vi "translate.vi"(8 "error in (no error)":errorcluster, 11 "ImagingModeDL090130Frame in":refnum<class "ImagingModeDL090130Frame.lvclass">=refnum) -> (0 "error out":errorcluster, 3 "ImagingModeDL090130Frame out":refnum<class "ImagingModeDL090130Frame.lvclass">)   [LabVIEW 2010, in "ImagingModeDL090130Frame.lvclass"]
uses:
  ImagingModeDL090130Frame.lvclass
  ScanHead/GenericScanHead/GenericScanHead/GenericScanHead.lvclass
  common/classes/GenericComponent/GenericComponent/GenericComponent.lvclass
  Adapter/GenericAdapter/GenericAdapter/GenericAdapter.lvclass
  ImagingModeDL090130Frame.lvclass/ImagingModeDL090130Frame.ctl
  common/classes/ErrorController/ErrorController/class_data.vi
  common/classes/ErrorController/ErrorController/ErrorController.lvclass
  Stage/GenericStage/GenericStage/GenericStage.lvclass
  Stage/GenericStage/GenericStage/translation_mode_enum.ctl
  GenericImagingMode/GenericImagingMode/GenericImagingMode.lvclass
  common/classes/SpaceVector/SpaceVector/SpaceVector.lvclass
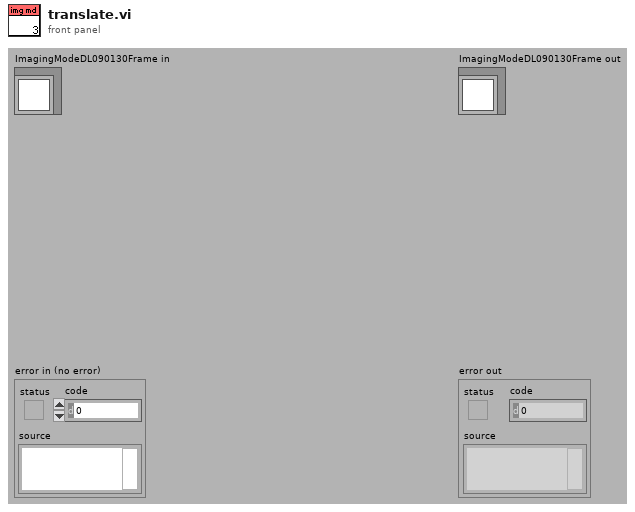
[diagram p1: front panel]
types:
  T1 = typedef "GenericStage.lvclass/translation_mode_enum.ctl" = enum16{"DON'T MOVE", "relative", "absolute"}
  T2 = typedef "ImagingModeDL090130Frame.lvclass/translation_mode_enum.ctl" = enum16{"scanHead", "stage"}
  T3 = typedef "GenericToplevelComponent.lvclass/common_trigger_enum.ctl" = enum16{"NULL", "initialise", "terminate", "fetch command", "fetch data", "attach observer", "register as observer", "detach observer", "acknowledge", "start", "stop", "sweep started", "sweep finished", "experiment started", "experiment stopped"}
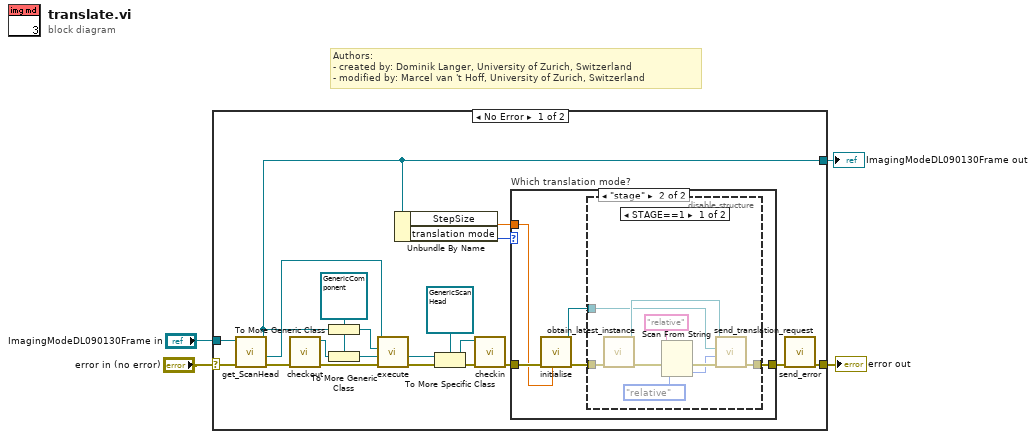
[diagram p0: block diagram]
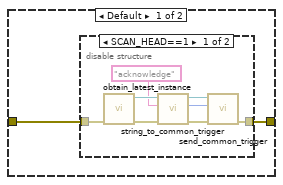
[diagram p2: hidden frame]
diagram:
  # "Authors: \n- created by: Dominik Langer, University of Zurich, Switzerland\n- modified by: Marcel van 't Hoff, University of Zurich, Switzerland"
  n1 = case shown="No Error" "error in (no error)" {
    selector: "error in (no error)" -> [w9 w52]
    tunnel: [w22 w52] -> w3
    tunnel: [w5 w51] -> w1
    tunnel: "ImagingModeDL090130Frame in" -> [w7 w51]
    frame No Error {
      w10 = refnum<class "GenericComponent.lvclass"> refnum ("GenericComponent.lvclass")
      n2 = call-dynamic "get_ScanHead.vi"("error in (no error)"=w9, "ScanModeDL090923Scaffold in"=w7) -> ("error out"=w8:errorcluster, "ScanHead adapter"=w6:refnum<class "GenericAdapter.lvclass">, "ScanModeDL090923Scaffold out"=w5:refnum<class "ImagingModeDL090130Frame.lvclass">)  [unwired: 4 in, 3 out]
      n3 = call "checkout.vi"("error in (no error)"=w8) -> ("error out"=w20:errorcluster, "GenericScanHead out"=w19:refnum<class "GenericScanHead.lvclass">)  [unwired: 9 in]
      n4 = To More Generic Class(target class=w10, reference=w5) -> (generic class reference=w17:refnum<class "GenericComponent.lvclass">)
      n5 = To More Generic Class(target class=w10, reference=w19) -> (generic class reference=w18:refnum<class "GenericComponent.lvclass">)
      n6 = call-dynamic "execute.vi"("error in (no error)"=w20, "B in"=w18, "A in"=w17, "GenericAdapter in"=w6) -> ("error out"=w15:errorcluster, "B out"=w16:refnum<class "GenericComponent.lvclass">)  [unwired: 4 in, 2 out]
      n7 = Unbundle By Name(w5) -> ("StepSize"=w24:dbl[unit], "translation mode"=w23:T2)
      n8 = To More Specific Class(target class=refnum<class "GenericScanHead.lvclass"> refnum ("GenericScanHead.lvclass"), reference=w16, error in=w15) -> (specific class reference=w12:refnum<class "GenericScanHead.lvclass">, error out=w14:errorcluster)
      n9 = call-dynamic "checkin.vi"("error in (no error)"=w14, "GenericScanHead in"=w12) -> ("error out"=w11:errorcluster)  [unwired: 8 in, 1 out]
      n10 = case "Which translation mode?" shown="\"stage\"" w23 {
        tunnel: w11 -> [w26 w39]
        tunnel: [w25 w40] -> w21
        tunnel: w24 -> [_ w37]
        frame Default {
          n11 = disable-structure shown="SCAN_HEAD==1" {
            disable-tunnel: w26 -> [w34 w35]
            disable-tunnel: [w33 w35] -> w25
            frame condition #0 {
              n12 = call "obtain_latest_instance.vi"("error in (no error)"=w34) -> ("error out"=w32:errorcluster, "GenericScanMode out"=w31:refnum<class "GenericImagingMode.lvclass">)  [unwired: 9 in]
              n13 = call-dynamic "string_to_common_trigger.vi"("error in (no error)"=w32, "trigger string"="acknowledge", "GenericToplevelComponent in"=w31) -> ("error out"=w29:errorcluster, "trigger"=w28:T3, "GenericToplevelComponent out"=w30:refnum<class "GenericImagingMode.lvclass">)  [unwired: 6 in]
              n14 = call-dynamic "send_common_trigger.vi"("error in (no error)"=w29, "trigger"=w28, "GenericToplevelComponent in"=w30) -> ("error out"=w33:errorcluster)  [unwired: 6 in, 2 out]
            }
            frame condition #1 (active) {
            }
          }
        }
        frame "stage" {
          n15 = call "initialise.vi"("z"=w37, "error in (no error)"=w39) -> ("error out"=w38:errorcluster, "SpaceVector out"=w36:refnum<class "SpaceVector.lvclass">)  [unwired: 8 in]
          n16 = disable-structure shown="STAGE==1" {
            disable-tunnel: w38 -> [w49 w50]
            disable-tunnel: [w48 w50] -> w40
            disable-tunnel: w36 -> [w46 _]
            frame condition #0 {
              n17 = call "obtain_latest_instance.vi"("error in (no error)"=w49) -> ("error out"=w45:errorcluster, "GenericStage out"=w47:refnum<class "GenericStage.lvclass">)  [unwired: 9 in]
              n18 = Scan From String(input string="relative", error in=w45, default 1=translation_mode_enum."relative" ("translation mode")) -> (error out=w44:errorcluster, output 1=w43:T1)  [unwired: 2 in, 2 out]
              n19 = call-dynamic "send_translation_request.vi"("error in (no error)"=w44, "translation mode"=w43, "translation vector"=w46, "GenericStage in"=w47) -> ("error out"=w48:errorcluster)  [unwired: 6 in, 1 out]
            }
            frame condition #1 (active) {
            }
          }
        }
      }
      n20 = call "send_error.vi"("error in (no error)"=w21) -> ("error out"=w22:errorcluster)  [unwired: 10 in]
    }
    frame Error {
    }
  }
  "error out" <- w3
  "ImagingModeDL090130Frame out" <- w1
